vi "POSITION ARMS MANUAL TELEOP.vi"(6 "IGNORE LIMITS?":bool, 7 "Use percent output?":bool=TRUE, 11 "Joystick values":T1(array[cluster])) -> ()   [LabVIEW 2020]
uses:
  <vilib>/Rock Robotics/WPI/ThirdParty/Phoenix-LabVIEW/Motor Controller/Controls/CTRE_Phoenix_MotorControl_ControlMode.ctl
  <vilib>/Rock Robotics/Network Tables/NT Read Boolean.vi
  Robot Global Data.vi
  <vilib>/Rock Robotics/Network Tables/NT Read Number.vi
  <vilib>/Rock Robotics/Network Tables/NT Write Number.vi
panel:
  in  "MIN JOYSTICK INPUT TO MOVE":dbl=0.1 format="%#_13g"
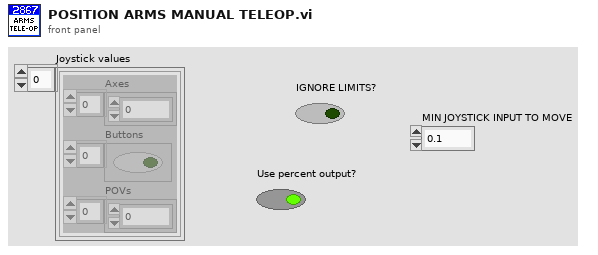
[diagram p1: front panel]
types:
  T1 = cluster{"Axes":dbl[], "Buttons":bool[], "POVs":i16[]}[]
  T2 = cluster{"Axes":dbl[], "Buttons":bool[], "POVs":i16[]}
  T3 = cluster{"MIN":dbl, "MAX":dbl, "convert climber inches to tics":dbl, "INITIALIZE":dbl}
  T4 = cluster{"MIN":dbl, "MAX":dbl, "convert arm inches to revs":dbl, "convert arm inches to degrees":dbl}
  T5 = typedef "CTRE_Phoenix_MotorControl_ControlMode.ctl" = u16
  T6 = typedef "WPI_MotorControlDeviceRef.ctl" = cluster{"DeviceStatus":errorcluster, "Type":T7, "PWM":cluster{"PWM Channel":T8, "DeadBand":T9}, "CAN":cluster{"Device Number":u8, "SetOutput VI Ref":variant, "GetOutput VI Ref":variant, "Enable VI Ref":variant, "Disable VI Ref":variant, "Data":variant}, "Invert":bool, "DIO PWM":cluster{"PWM \"Enable\" Channel":T8, "DIOChannel":T10, "PWM Rate":dbl}}
  T7 = typedef "WPI_MotorControlType.ctl" = enum16{"PWM", "CAN", "DIO PWM"}
  T8 = typedef "FPGA_DIOPWMChannel.ctl" = enum8{"PWM 0", "PWM 1", "PWM 2", "PWM 3", "PWM 4", "PWM 5", "PWM 6", "PWM 7", "PWM 8", "PWM 9", "PWM MXP 0", "PWM MXP 1", "PWM MXP 2", "PWM MXP 3", "PWM MXP 4", "PWM MXP 5", "PWM MXP 6", "PWM MXP 7", "PWM MXP 8", "PWM MXP 9", "Invalid"}
  T9 = typedef "WPI_PWMDeadband.ctl" = cluster{"Name":string, "maxPositivePwm":i32, "minPositivePwm":i32, "centerPwm":i32, "maxNegativePwm":i32, "minNegativePwm":i32, "angularRange":u16}
  T10 = typedef "FPGA_DIOChannel.ctl" = enum8{"DIO 0", "DIO 1", "DIO 2", "DIO 3", "DIO 4", "DIO 5", "DIO 6", "DIO 7", "DIO 8", "DIO 9", "DIO MXP 0", "DIO MXP 1", "DIO MXP 2", "DIO MXP 3", "DIO MXP 4", "DIO MXP 5", "DIO MXP 6", "DIO MXP 7", "DIO MXP 8", "DIO MXP 9", "DIO MXP 10", "DIO MXP 11", "DIO MXP 12", "DIO MXP 13", "DIO MXP 14", "DIO MXP 15", "SPI Port CS1", "SPI Port CS2", "SPI Port CS3", "SPI Port MISO", "SPI Port MOSI", "Invalid"}
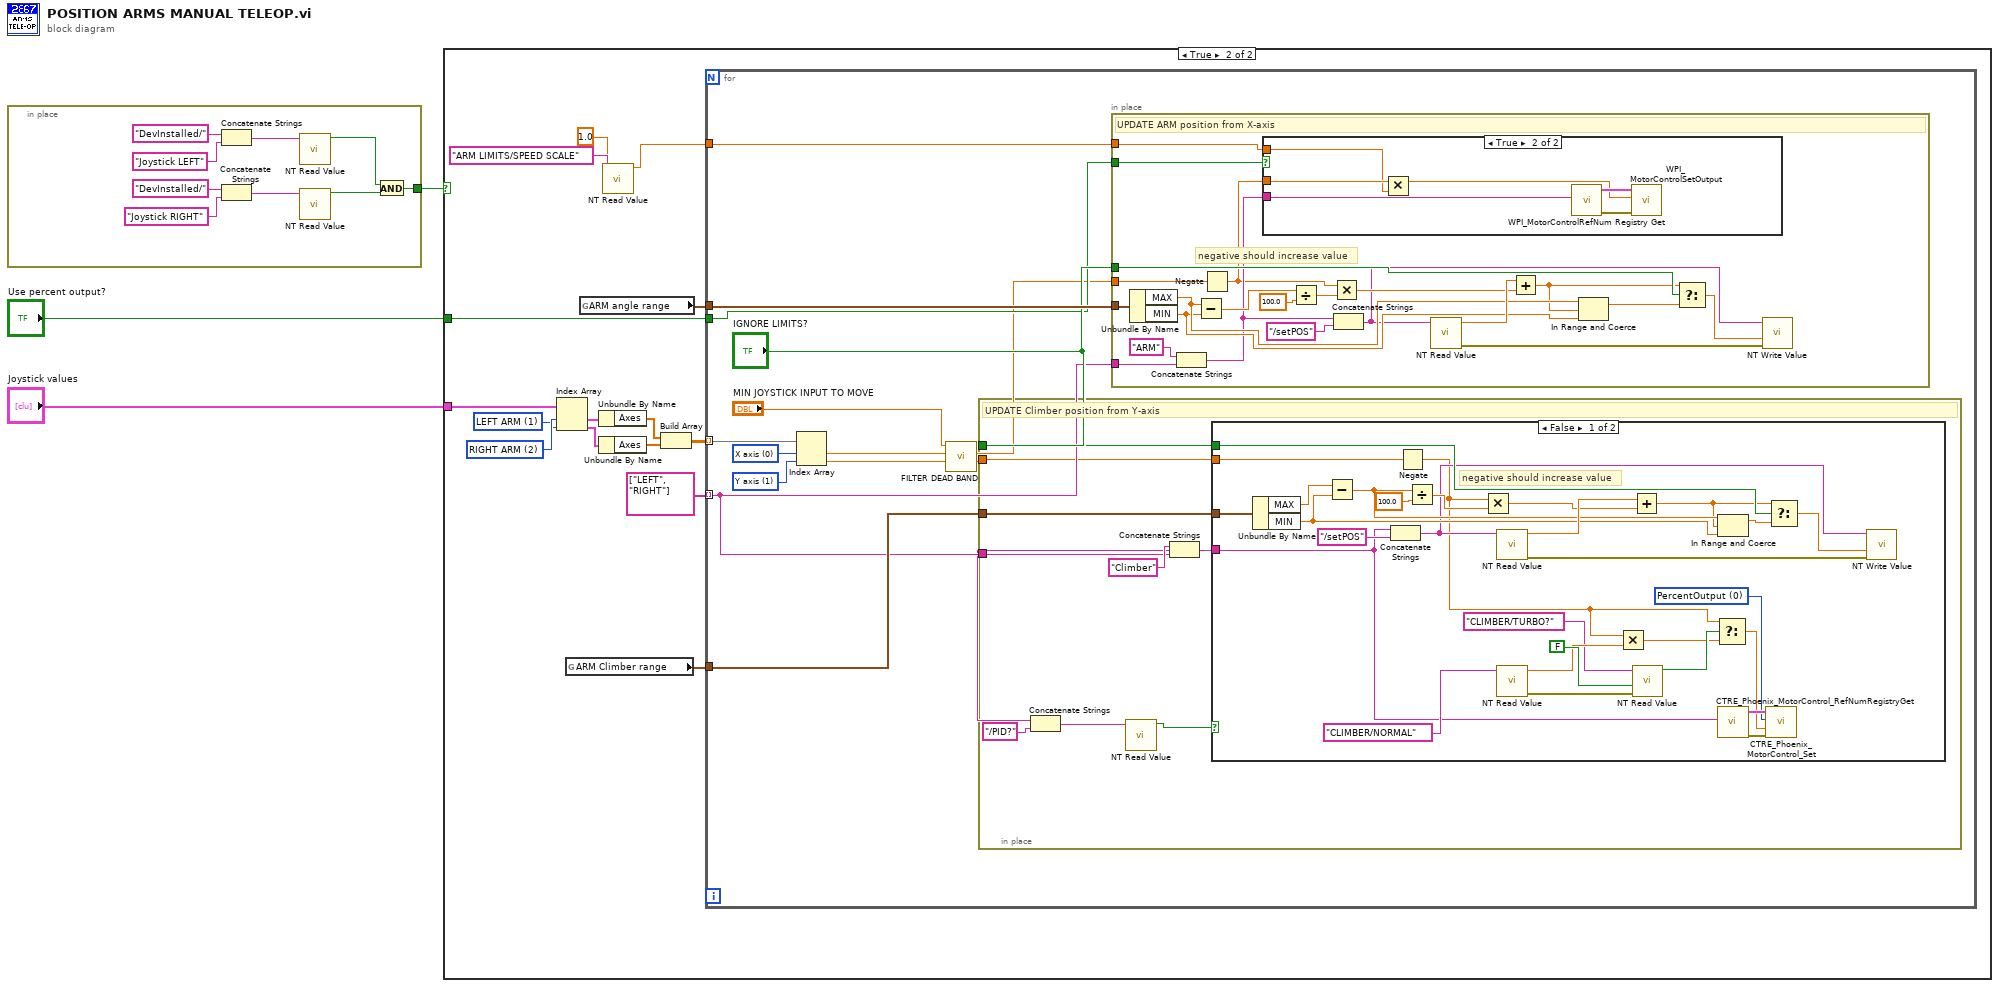
[diagram p0: block diagram]
diagram:
  n1 = in-place {
    in-place-border: [w4] -> w2
    n2 = Concatenate Strings("DevInstalled/" ("Name"), "Joystick LEFT" ("Name")) -> (w12:string)
    n3 = Concatenate Strings("DevInstalled/" ("Name"), "Joystick RIGHT" ("Name")) -> (w9:string)
    n4 = call-poly <vilib>:"NT Read Value.vi"("Name"=w12) -> ("Boolean"=w5:bool)  [unwired: 9 in, 1 out]
    n5 = call-poly <vilib>:"NT Read Value.vi"("Name"=w9) -> ("Boolean"=w6:bool)  [unwired: 9 in, 1 out]
    n6 = And(x=w5, y=w6) -> (x .and. y?=w4:bool)
  }
  n7 = case shown="True" w2 {
    tunnel: "Joystick values" -> [_ w24]
    tunnel: "Use percent output?" -> [_ w18]
    frame False {
    }
    frame True {
      w17 = u16 2 items=["RIGHT TANK (default)", "LEFT ARM", "RIGHT ARM", "LEFT TANK DRIVE"] ("Joysticks")
      w16 = u16 1 items=["RIGHT TANK (default)", "LEFT ARM", "RIGHT ARM", "LEFT TANK DRIVE"] ("Joysticks")
      n8 = Index Array(array=w24, index #1=w17, index #2=w16) -> (element #1=w23:T2, element #2=w20:T2)
      n9 = global read "Robot Global Data.vi" "ARM Climber range"() -> (w26:T3)
      n10 = global read "Robot Global Data.vi" "ARM angle range"() -> (w25:T4)
      n11 = Unbundle By Name(w23) -> ("Axes"=w21:dbl[])
      n12 = Unbundle By Name(w20) -> ("Axes"=w19:dbl[])
      n13 = call-poly <vilib>:"NT Read Value.vi"("Default Value"=1.0, "Name"="ARM LIMITS/SPEED SCALE") -> ("Numeric"=w14:dbl)  [unwired: 8 in, 1 out]
      n14 = Build Array(w21, w19) -> (w22:dbl[][])
      n15 = for {
        tunnel: string[] ["LEFT", "RIGHT"] -> [w29] mode=indexing
        tunnel: w22 -> [w41] mode=indexing
        tunnel: w26 -> [w38]
        tunnel: w25 -> [w37]
        tunnel: w18 -> [w33]
        tunnel: w14 -> [w28]
        w35 = u16 1 items=["X axis", "Y axis", "Z axis"] ("AXIS VALUES")
        w36 = u16 0 items=["X axis", "Y axis", "Z axis"] ("AXIS VALUES")
        n16 = Index Array(array=w41, index #1=w36, index #2=w35) -> (element #1=w40:dbl, element #2=w39:dbl)
        n17 = call "FILTER DEAD BAND.vi"("Joystick value in 2"=w39, "Joystick value in"=w40, "dead band%"="MIN JOYSTICK INPUT TO MOVE") -> ("Joystick value out 2"=w32:dbl, "Joystick value out"=w31:dbl)  [unwired: 7 in]
        n18 = in-place {
          in-place-border: w29 -> [w72]
          in-place-border: w32 -> [w78]
          in-place-border: w38 -> [w77]
          in-place-border: "IGNORE LIMITS?" -> [w76]
          # "UPDATE Climber position from Y-axis"
          n19 = Concatenate Strings("Climber" ("string"), w72) -> (w71:string)
          n20 = Concatenate Strings(w71, "/PID?" ("string")) -> (w75:string)
          n21 = call-poly <vilib>:"NT Read Value.vi"("Name"=w75) -> ("Boolean"=w70:bool)  [unwired: 9 in, 1 out]
          n22 = case shown="False" w70 {
            tunnel: w78 -> [w104 _]
            tunnel: w77 -> [w101 _]
            tunnel: w76 -> [w95 _]
            tunnel: w71 -> [w79 _]
            frame False {
              w88 = T5 0 items=["PercentOutput"=0, "Position"=1, "Velocity"=2, "Current"=3, "Follower"=5, "MotionProfile"=6, "MotionMagic"=7, "MotionProfileArc"=10, "Disabled"=15] ("Control Mode")
              # "negative should increase value"
              n23 = Unbundle By Name(w101) -> ("MAX"=w100:dbl, "MIN"=w98:dbl)
              n24 = Subtract(x=w100, y=w98) -> (x-y=w99:dbl)
              n25 = Concatenate Strings(w79, "/setPOS" ("string")) -> (w93:string)
              n26 = Negate(x=w104) -> (-x=w91:dbl)
              n27 = Divide(x=w99, y=100.0) -> (x/y=w103:dbl)
              n28 = Multiply(x=w91, y=w103) -> (x*y=w105:dbl)
              n29 = call-poly <vilib>:"NT Read Value.vi"("Name"=w93) -> ("error out"=w107:errorcluster, "Numeric"=w106:dbl)  [unwired: 9 in]
              n30 = call-poly <vilib>:"NT Read Value.vi"("Name"="CLIMBER/NORMAL") -> ("error out"=w87:errorcluster, "Numeric"=w82:dbl)  [unwired: 9 in]
              n31 = Multiply(x=w91, y=w82) -> (x*y=w83:dbl)
              n32 = Add(x=w106, y=w105) -> (x+y=w94:dbl)
              n33 = call-poly <vilib>:"NT Read Value.vi"("error in"=w87, "Default Value"=FALSE, "Name"="CLIMBER/TURBO?") -> ("Boolean"=w84:bool)  [unwired: 7 in, 1 out]
              n34 = Select(t=w91, s=w84, f=w83) -> (s? t:f=w85:dbl)
              n35 = In Range and Coerce(upper limit=w99, x=w94, lower limit=w98) -> (coerced(x)=w96:dbl)  [unwired: 1 out]
              n36 = call <vilib>:"CTRE_Phoenix_MotorControl_RefNumRegistryGet.vi"("refnum name"=w79) -> ("error out"=w90:errorcluster, "PhoenixMotorControlDevRef"=w89:T6)  [unwired: 9 in]
              n37 = call <vilib>:"CTRE_Phoenix_MotorControl_Set.vi"("error in (no error)"=w90, "Output"=w85, "Control Mode"=w88, "PhoenixMotorControlDevRef"=w89) -> ()  [unwired: 6 in, 2 out]
              n38 = Select(t=w94, s=w95, f=w96) -> (s? t:f=w97:dbl)
              n39 = call-poly <vilib>:"NT Write Value.vi"("error in"=w107, "Numeric"=w97, "Name"=w93) -> ()  [unwired: 8 in, 1 out]
            }
            frame True {
            }
          }
        }
        n40 = in-place {
          in-place-border: w29 -> [w63]
          in-place-border: w31 -> [w58]
          in-place-border: w37 -> [w54]
          in-place-border: "IGNORE LIMITS?" -> [w49]
          in-place-border: w33 -> [w45]
          in-place-border: w28 -> [w42]
          # "negative should increase value"
          # "UPDATE ARM position from X-axis"
          n41 = Unbundle By Name(w54) -> ("MAX"=w53:dbl, "MIN"=w52:dbl)
          n42 = Concatenate Strings("ARM" ("string"), w63) -> (w44:string)
          n43 = Subtract(x=w53, y=w52) -> (x-y=w55:dbl)
          n44 = Negate(x=w58) -> (-x=w43:dbl)
          n45 = case shown="True" w45 {
            tunnel: w44 -> [_ w69]
            tunnel: w43 -> [_ w66]
            tunnel: w42 -> [_ w64]
            frame False {
            }
            frame True {
              n46 = Multiply(x=w66, y=w64) -> (x*y=w65:dbl)
              n47 = call <vilib>:"WPI_MotorControlRefNum Registry Get.vi"("refnum name"=w69) -> ("error out"=w68:errorcluster, "MotorControlDevRef"=w67:T6)  [unwired: 9 in]
              n48 = call <vilib>:"WPI_MotorControlSetOutput.vi"("error in (no error)"=w68, "Output"=w65, "MotorControlDevRef"=w67) -> ()  [unwired: 6 in, 3 out]
            }
          }
          n49 = Divide(x=w55, y=100.0) -> (x/y=w57:dbl)
          n50 = Multiply(x=w43, y=w57) -> (x*y=w59:dbl)
          n51 = Concatenate Strings(w44, "/setPOS" ("string")) -> (w47:string)
          n52 = call-poly <vilib>:"NT Read Value.vi"("Name"=w47) -> ("error out"=w61:errorcluster, "Numeric"=w60:dbl)  [unwired: 9 in]
          n53 = Add(x=w60, y=w59) -> (x+y=w48:dbl)
          n54 = In Range and Coerce(upper limit=w53, x=w48, lower limit=w52) -> (coerced(x)=w50:dbl)  [unwired: 1 out]
          n55 = Select(t=w48, s=w49, f=w50) -> (s? t:f=w51:dbl)
          n56 = call-poly <vilib>:"NT Write Value.vi"("error in"=w61, "Numeric"=w51, "Name"=w47) -> ()  [unwired: 8 in, 1 out]
        }
      }
    }
  }
